vi "adam-ALL-IOs-panel-no-references.vi"(0 "VISA Refnum in":refnum<visa-resource-name>, 1 "ADAM-5000-data-current":T3, 3 "Digital Outputs":T4, 4 "Analog Outputs":T6, 5 "error in (no error)":errorcluster, 6 "Module Type":T10(ring), 7 "chassis-slot":i32=5, 9 "cmd-response in":T1, 10 "Chassis Settings":T8) -> (12 "slot: x":T9, 13 "output indicator":cluster{"cmd aknowledged":bool, "Sampling":bool}, 14 "VISA Refnum out":refnum<visa-resource-name>, 15 "ADAM-5000-data-new":T3, 18 "cmd-response out":T1, 19 "error out":errorcluster)   [LabVIEW 2024]
uses:
  controls/digital-output-cluster.ctl
  controls/digitial-input-cluster.ctl
  controls/analog-input-cluster.ctl
  controls/thermocouple-input-cluster.ctl
  controls/adam-module-select-tab.ctl
  controls/adam-5000-serial-settings.ctl
  controls/analog-output-cluster.ctl
  controls/adam-5000-all-module-datas.ctl
  controls/adam-5000-cmd-response.ctl
panel:
  out "Analog Inputs":T2
  out "Digital Inputs":T5
  out "Thermocouple Inputs (degC)":T7
  # "No References for Sampling and Ack Indicators -\nSimplifies requirements to implement"
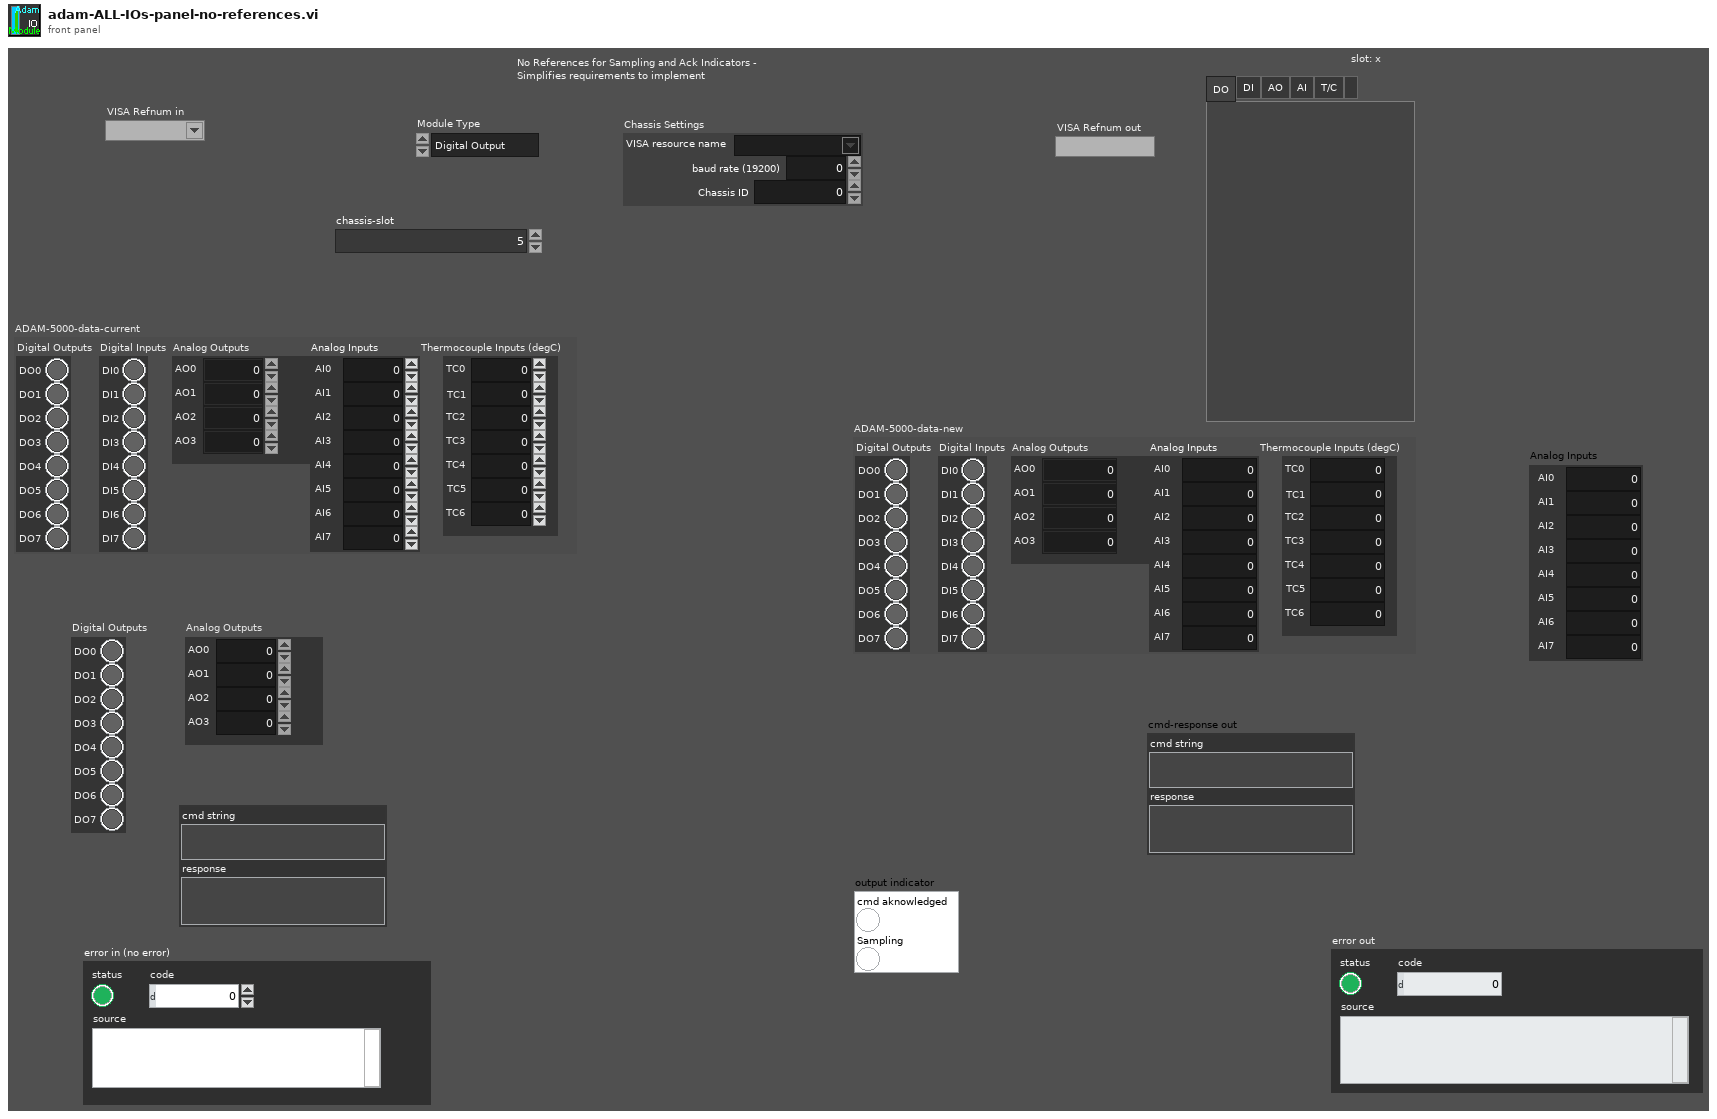
[diagram p1: front panel]
types:
  T1 = typedef "adam-5000-cmd-response.ctl" = cluster{"cmd string":string, "response":string}
  T2 = typedef "analog-input-cluster.ctl" = cluster{"AI0":dbl, "AI1":dbl, "AI2":dbl, "AI3":dbl, "AI4":dbl, "AI5":dbl, "AI6":dbl, "AI7":dbl}
  T3 = typedef "adam-5000-all-module-datas.ctl" = cluster{"Digital Outputs":T4, "Digital Inputs":T5, "Analog Outputs":T6, "Analog Inputs":T2, "Thermocouple Inputs (degC)":T7}
  T4 = typedef "digital-output-cluster.ctl" = cluster{"DO0":bool, "DO1":bool, "DO2":bool, "DO3":bool, "DO4":bool, "DO5":bool, "DO6":bool, "DO7":bool}
  T5 = typedef "digitial-input-cluster.ctl" = cluster{"DI0":bool, "DI1":bool, "DI2":bool, "DI3":bool, "DI4":bool, "DI5":bool, "DI6":bool, "DI7":bool}
  T6 = typedef "analog-output-cluster.ctl" = cluster{"AO0":dbl, "AO1":dbl, "AO2":dbl, "AO3":dbl}
  T7 = typedef "thermocouple-input-cluster.ctl" = cluster{"TC0":dbl, "TC1":dbl, "TC2":dbl, "TC3":dbl, "TC4":dbl, "TC5":dbl, "TC6":dbl}
  T8 = typedef "adam-5000-serial-settings.ctl" = cluster{"VISA resource name":refnum<visa-resource-name>, "baud rate (19200)":u32, "Chassis ID":u8}
  T9 = typedef "adam-module-select-tab.ctl" = enum32{"DO", "DI", "AO", "AI", "T/C", ""}
  T10 = enum16{"Digital Output", "Digital Input", "Analog Output", "Analog Input", "Thermocouple", "Power Relay", "empty"}
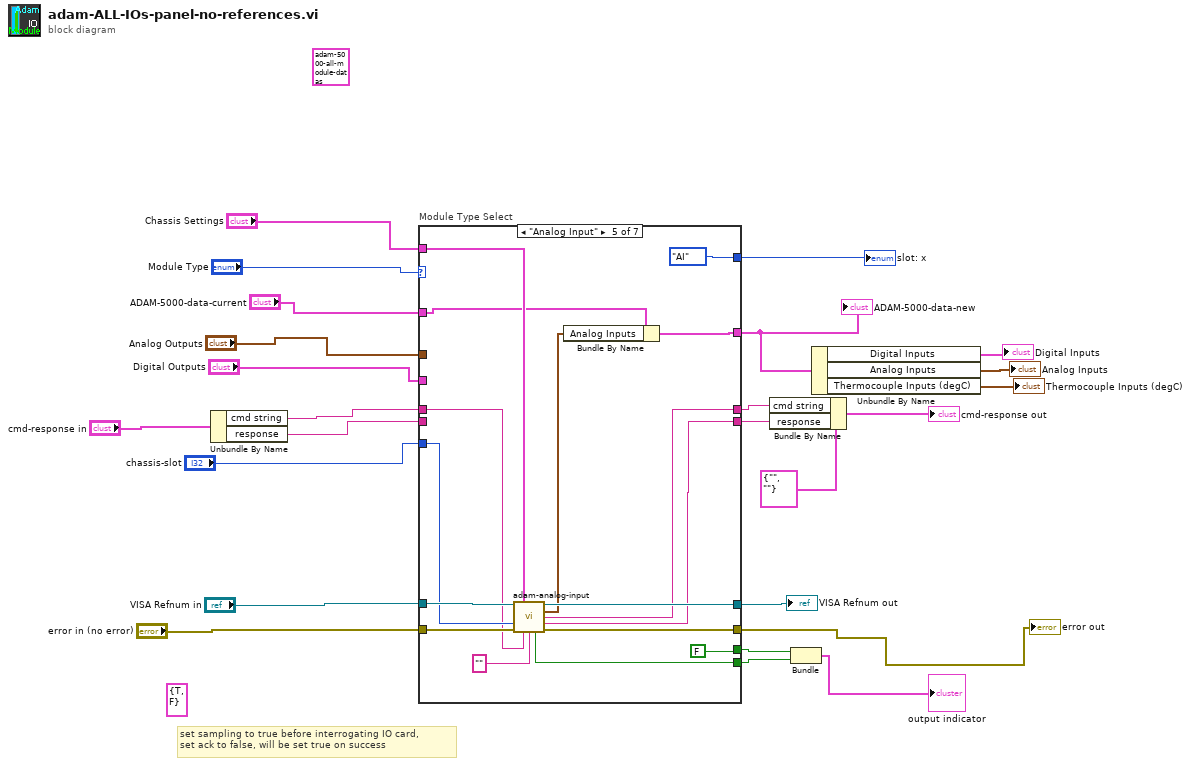
[diagram p0: block diagram]
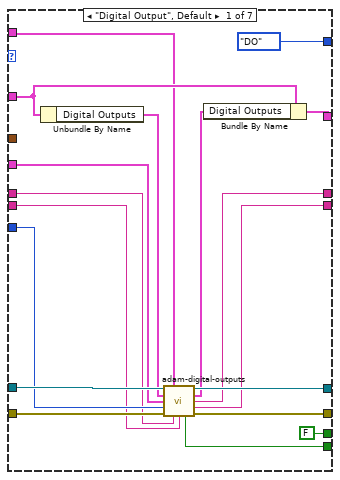
[diagram p2: hidden frame]
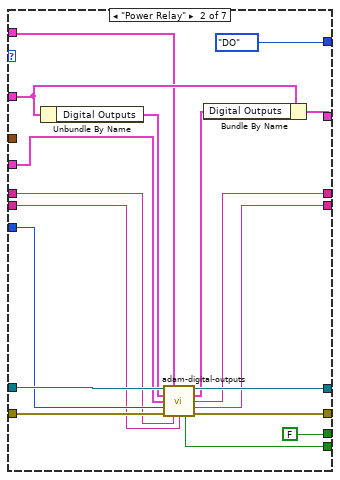
[diagram p3: hidden frame]
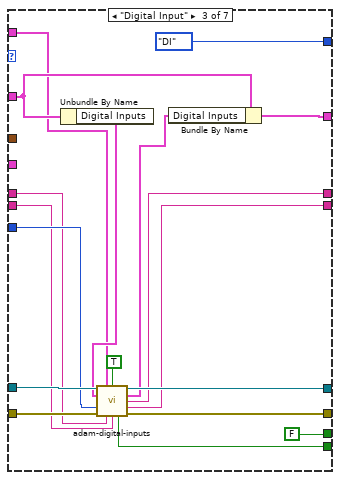
[diagram p4: hidden frame]
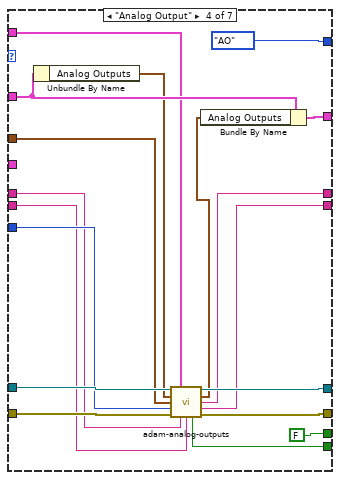
[diagram p5: hidden frame]
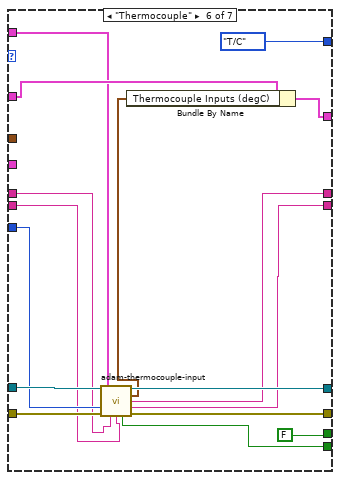
[diagram p6: hidden frame]
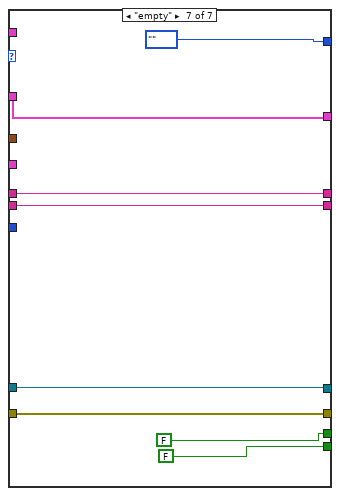
[diagram p7: hidden frame]
diagram:
  (unwired) cluster{"Sampling":bool, "Ack":bool} {"Sampling"=TRUE, "Ack"=FALSE} ("Value")
  (unwired) T3 {"Digital Outputs"={"DO0"=FALSE, "DO1"=FALSE, "DO2"=FALSE, "DO3"=FALSE, "DO4"=FALSE, "DO5"=FALSE, "DO6"=FALSE, "DO7"=FALSE}, "Digital Inputs"={"DI0"=FALSE, "DI1"=FALSE, "DI2"=FALSE, "DI3"=FALSE, "DI4"=FALSE, "DI5"=FALSE, "DI6"=FALSE, "DI7"=FALSE}, "Analog Outputs"={"AO0"=0.0, "AO1"=0.0, "AO2"=0.0, "AO3"=0.0}, "Analog Inputs"={"AI0"=0.0, "AI1"=0.0, "AI2"=0.0, "AI3"=0.0, "AI4"=0.0, "AI5"=0.0, "AI6"=0.0, "AI7"=0.0}, "Thermocouple Inputs (degC)"={"TC0"=0.0, "TC1"=0.0, "TC2"=0.0, "TC3"=0.0, "TC4"=0.0, "TC5"=0.0, "TC6"=0.0}} ("ADAM-5000-data-typedefs")
  # "set sampling to true before interrogating IO card,\nset ack to false, will be set true on success"
  n1 = Unbundle By Name("cmd-response in") -> ("cmd string"=w13:string, "response"=w14:string)
  n2 = case "Module Type Select" shown="\"Analog Input\"" "Module Type" {
    tunnel: "ADAM-5000-data-current" -> [w41 w59 w73 w96 w106 w129 w130]
    tunnel: [adam-module-select-tab."DO" ("slot: 0") adam-module-select-tab."DO" ("slot: 0") adam-module-select-tab."DI" ("slot: 0") adam-module-select-tab."AO" ("slot: 0") adam-module-select-tab."AI" ("slot: 0") adam-module-select-tab."T/C" ("slot: 0") adam-module-select-tab."" ("slot: 0")] -> w20
    tunnel: [w42 w60 w78 w95 w105 w128 w130] -> w18
    tunnel: "Chassis Settings" -> [w31 w49 w66 w87 w113 w122 _]
    tunnel: "chassis-slot" -> [w34 w52 w71 w88 w108 w121 _]
    tunnel: "VISA Refnum in" -> [w40 w58 w77 w92 w112 w126 w131]
    tunnel: "error in (no error)" -> [w39 w57 w76 w94 w111 w125 w132]
    tunnel: [w38 w56 w75 w93 w110 w124 w132] -> w2
    tunnel: [w37 w55 w74 w91 w109 w123 w131] -> w22
    tunnel: [w32 w50 w67 w85 w107 w117 w134] -> w7
    tunnel: w14 -> [w29 w47 w69 w84 _ w119 w134]
    tunnel: w13 -> [w30 w48 w70 w83 w102 w120 w135]
    tunnel: [w27 w44 w62 w80 w98 w114 FALSE ("Sampling")] -> w11
    tunnel: [w33 w51 w68 w86 w103 w118 w135] -> w8
    tunnel: [FALSE ("cmd aknowledged") FALSE ("Sampling") FALSE ("Sampling") FALSE ("Sampling") FALSE ("Sampling") FALSE ("Sampling") FALSE ("cmd aknowledged")] -> w12
    tunnel: "Digital Outputs" -> [w28 w46 _ _ _ _ _]
    tunnel: "Analog Outputs" -> [_ _ _ w82 _ _ _]
    frame "Digital Output", Default {
      n3 = Unbundle By Name(w41) -> ("Digital Outputs"=w36:T4)
      n4 = call "adam-digital-outputs.vi"("VISA Refnum in"=w40, "Chassis Settings"=w31, "Current DO State"=w36, "DO Control"=w28, "chassis-slot"=w34, "error in (no error)"=w39, "cmd-in"=w30, "ack char"=w29) -> ("VISA Refnum out"=w37:refnum<visa-resource-name>, "New DO State"=w35:T4, "cmd-out"=w33:string, "acknowledge char"=w32:string, "cmd aknowledged"=w27:bool, "error out"=w38:errorcluster)  [unwired: 2 in]
      n5 = Bundle By Name(cluster=w41, "Digital Outputs"=w35) -> (w42:T3)
    }
    frame "Power Relay" {
      n6 = Unbundle By Name(w59) -> ("Digital Outputs"=w54:T4)
      n7 = call "adam-digital-outputs.vi"("VISA Refnum in"=w58, "Chassis Settings"=w49, "Current DO State"=w54, "DO Control"=w46, "chassis-slot"=w52, "error in (no error)"=w57, "cmd-in"=w48, "ack char"=w47) -> ("VISA Refnum out"=w55:refnum<visa-resource-name>, "New DO State"=w53:T4, "cmd-out"=w51:string, "acknowledge char"=w50:string, "cmd aknowledged"=w44:bool, "error out"=w56:errorcluster)  [unwired: 2 in]
      n8 = Bundle By Name(cluster=w59, "Digital Outputs"=w53) -> (w60:T3)
    }
    frame "Digital Input" {
      n9 = Unbundle By Name(w73) -> ("Digital Inputs"=w72:T5)
      n10 = call "adam-digital-inputs.vi"("VISA Refnum in"=w77, "Chassis Settings"=w66, "sample?"=TRUE, "Current DI State"=w72, "chassis-slot"=w71, "error in (no error)"=w76, "cmd-in"=w70, "ack char"=w69) -> ("VISA Refnum out"=w74:refnum<visa-resource-name>, "New DI State"=w64:T5, "cmd-out"=w68:string, "acknowledge char"=w67:string, "cmd aknowledged"=w62:bool, "error out"=w75:errorcluster)  [unwired: 2 in]
      n11 = Bundle By Name(cluster=w73, "Digital Inputs"=w64) -> (w78:T3)
    }
    frame "Analog Output" {
      n12 = Unbundle By Name(w96) -> ("Analog Outputs"=w90:T6)
      n13 = call "adam-analog-outputs.vi"("VISA Refnum in"=w92, "Chassis Settings"=w87, "Current AO States"=w90, "Analog Outputs in"=w82, "chassis-slot"=w88, "error in (no error)"=w94, "Last cmd"=w83, "last ack message"=w84) -> ("VISA Refnum out"=w91:refnum<visa-resource-name>, "Analog Outputs out"=w89:T6, "cmd output"=w86:string, "ack message"=w85:string, "cmd aknowledged"=w80:bool, "error out"=w93:errorcluster)  [unwired: 2 in]
      n14 = Bundle By Name(cluster=w96, "Analog Outputs"=w89) -> (w95:T3)
    }
    frame "Analog Input" {
      n15 = call "adam-analog-input.vi"("VISA Refnum in"=w112, "Chassis Settings"=w113, "chassis-slot"=w108, "error in (no error)"=w111, "last cmd in"=w102, "last read buffer"="") -> ("VISA Refnum out"=w109:refnum<visa-resource-name>, "Analog Inputs"=w101:T2, "cmd out"=w103:string, "read-buffer out"=w107:string, "cmd aknowledged"=w98:bool, "error out"=w110:errorcluster)  [unwired: 4 in]
      n16 = Bundle By Name(cluster=w106, "Analog Inputs"=w101) -> (w105:T3)
    }
    frame "Thermocouple" {
      n17 = call "adam-thermocouple-input.vi"("VISA Refnum in"=w126, "Chassis Settings"=w122, "chassis-slot"=w121, "error in (no error)"=w125, "last cmd in"=w120, "last read buffer"=w119) -> ("VISA Refnum out"=w123:refnum<visa-resource-name>, "Thermocouple Inputs (degC)"=w116:T7, "cmd out"=w118:string, "read-buffer out"=w117:string, "cmd aknowledged"=w114:bool, "error out"=w124:errorcluster)  [unwired: 4 in]
      n18 = Bundle By Name(cluster=w129, "Thermocouple Inputs (degC)"=w116) -> (w128:T3)
    }
    frame "empty" {
    }
  }
  "slot: x" <- w20
  "VISA Refnum out" <- w22
  "error out" <- w2
  "ADAM-5000-data-new" <- w18
  n19 = Bundle By Name(cluster=T1 {"cmd string"="", "response"=""} ("cmd-response:0"), "cmd string"=w8, "response"=w7) -> (→"cmd-response out":T1)
  n20 = Bundle("cmd aknowledged"=w12, "Sampling"=w11) -> (→"output indicator":cluster{"cmd aknowledged":bool, "Sampling":bool})  [unwired: 1 in]
  n21 = Unbundle By Name(w18) -> ("Digital Inputs"=→"Digital Inputs":T5, "Analog Inputs"=→"Analog Inputs":T2, "Thermocouple Inputs (degC)"=→"Thermocouple Inputs (degC)":T7)
